vi "post-suite action.vi"(8 "error in (no error)":errorcluster, 11 "Test Runner.JUnit in":refnum<class "Test Runner.JUnit.lvclass">) -> (0 "error out":errorcluster, 3 "Test Runner.JUnit out":refnum<class "Test Runner.JUnit.lvclass">)   [LabVIEW 2013, in "Test Runner.JUnit.lvclass"]
uses:
  Test Runner.JUnit.lvclass
  classes/Test Runner/Test Runner.lvclass
  Test Runner.JUnit.lvclass/Test Runner.JUnit.ctl
  <vilib>/regexp/Match Regular Expression.xnode
  classes/Test/Test.lvclass
  classes/Assert/Assert.lvclass
panel:
  out "substring 2":string
  out "substring":string
  out "text":string
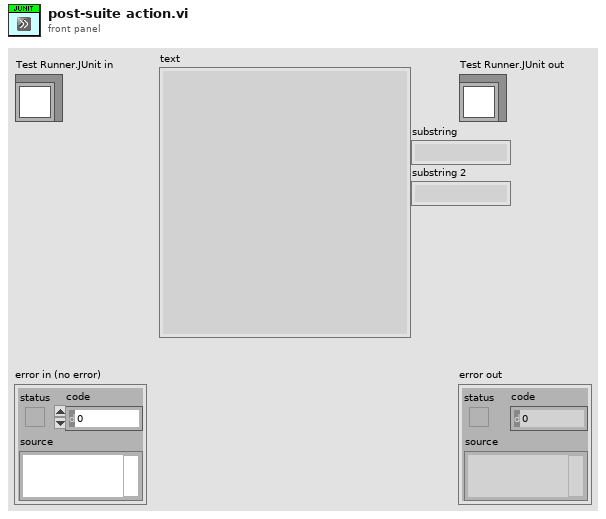
[diagram p1: front panel]
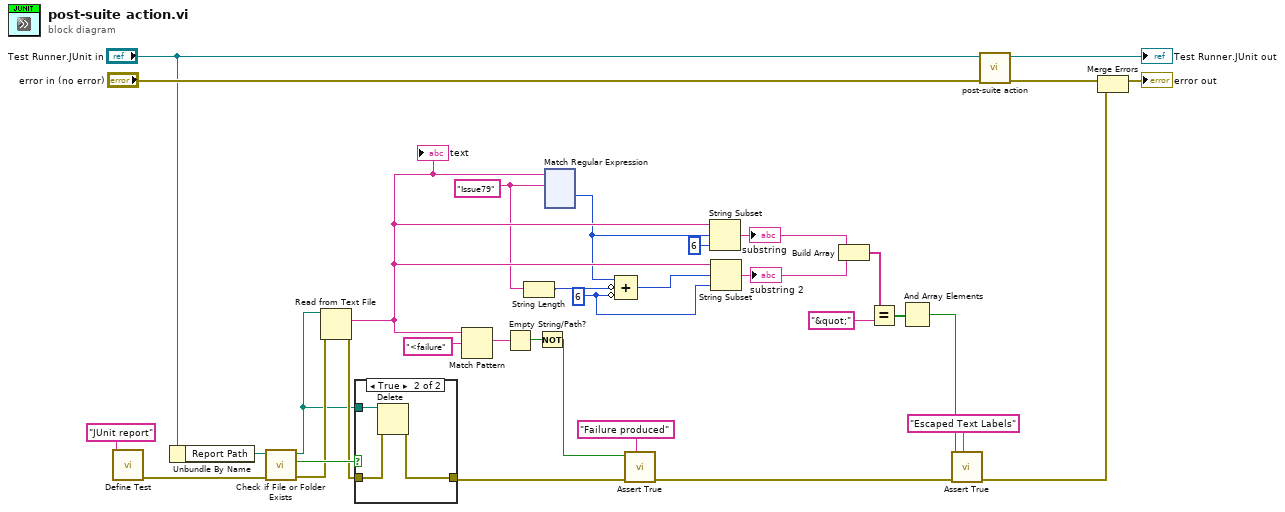
[diagram p0: block diagram]
diagram:
  w1 = 6 ("length (rest)")
  w14 = "Issue79" ("regular expression")
  n1 = call "Define Test.vi"("Label (VI Title)"="JUnit report") -> ("error out"=w24:errorcluster)  [unwired: 10 in]
  n2 = Unbundle By Name("Test Runner.JUnit in") -> ("Report Path"=w25:path)
  n3 = call <vilib>:"Check if File or Folder Exists.vi"("error in (no error)"=w24, "path"=w25) -> ("error out"=w31:errorcluster, "file or folder exists?"=w32:bool, "dup path"=w29:path)  [unwired: 7 in]
  n4 = Read from Text File(file (use dialog)=w29, error in=w31) -> (text=w15:string, error out=w30:errorcluster)  [unwired: 2 in, 2 out]
  "text" <- w15
  n5 = case shown="True" w32 {
    tunnel: w29 -> [_ w38]
    tunnel: w30 -> [w35 w37]
    tunnel: [w35 w36] -> w21
    frame False {
    }
    frame True {
      n6 = Delete(path (use dialog)=w38, error in=w37) -> (error out=w36:errorcluster)  [unwired: 3 in, 2 out]
    }
  }
  n7 = Match Pattern(string=w15, regular expression="<failure") -> (match substring=w27:string)  [unwired: 1 in, 3 out]
  n8 = Empty String/Path?(string/path=w27) -> (empty?=w26:bool)
  n9 = String Length(string=w14) -> (length=w12:i32)
  n10 = Not(x=w26) -> (.not. x?=w22:bool)
  n11 = xnode "Match Regular Expression"("input string"=w15, "regular expression"=w14) -> ("offset past match"=w13:i32)  [unwired: 4 in, 4 out]
  n12 = Compound Arithmetic op=ADD(w13, invert w12, invert w1) -> (w11:i32)
  n13 = call "Assert True.vi"("Label"="Failure produced", "error in (no error)"=w21, "True?"=w22) -> ("error out"=w8:errorcluster)  [unwired: 8 in]
  n14 = String Subset(string=w15, offset (0)=w13, length (rest)=6 ("length (rest)")) -> (substring=w10:string)
  "substring" <- w10
  n15 = String Subset(string=w15, offset (0)=w11, length (rest)=w1) -> (substring=w9:string)
  "substring 2" <- w9
  n16 = Build Array(w10, w9) -> (w6:string[])
  n17 = Equal?(x=w6, y="&quot;" ("regular expression")) -> (x = y?=w4:bool[])
  n18 = And Array Elements(Boolean array=w4) -> (logical AND=w3:bool)
  n19 = call "Assert True.vi"("Label"="Escaped Text Labels", "error in (no error)"=w8, "True?"=w3) -> ("error out"=w7:errorcluster)  [unwired: 8 in]
  n20 = call-parent "post-suite action.vi"("error in (no error)"="error in (no error)", "Test Runner in"="Test Runner.JUnit in") -> ("error out"=w20:errorcluster, "Test Runner out"=→"Test Runner.JUnit out":refnum<class "Test Runner.JUnit.lvclass">)  [unwired: 8 in]
  n21 = Merge Errors(w20, w7) -> (→"error out":errorcluster)
